vi "check_rs.vi"() -> ()   [LabVIEW 2013]
panel:
  in  "R&S address":string="29"
  out "address 2":string
  in  "amplitude (mV)":i32=10
  in  "modulation (kHz)":i32=100
  in  "center frequency (MHz)":dbl=32.7
  in  "exit":bool
  in  "rs_set":bool
  in  "rs_off":bool
  in  "rs_on":bool
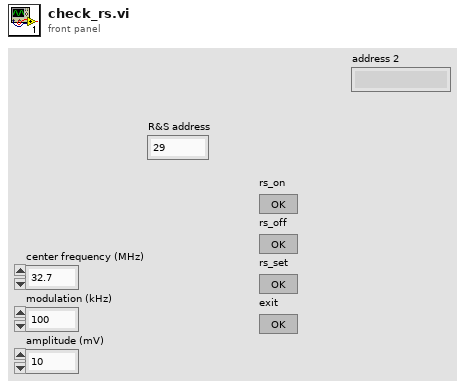
[diagram p1: front panel]
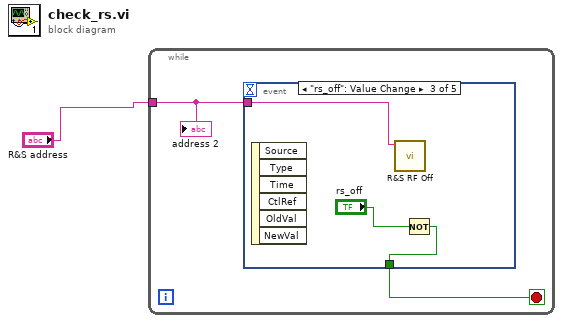
[diagram p0: block diagram]
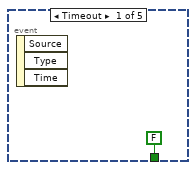
[diagram p2: hidden frame]
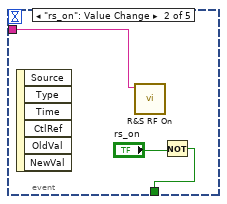
[diagram p3: hidden frame]
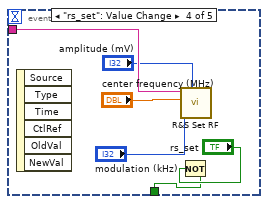
[diagram p4: hidden frame]
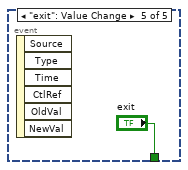
[diagram p5: hidden frame]
diagram:
  n1 = while {
    tunnel: "R&S address" -> [w2]
    stop <- w3 stop-if-true
    n2 = event shown="[2] \"rs_off\": Value Change" {
      selector: _ -> [_ _ _ _ _]
      dyn-events: _ -> [_ _ _ _ _]
      timeout: _ -> [_ _ _ _ _]
      tunnel: [FALSE ("exit") w5 w8 w11 "exit"] -> w3
      tunnel: w2 -> [_ w7 w10 w16 _]
      event Timeout {
        n3 = event-data() -> ()  [unwired: 1 in, 3 out]
      }
      event "rs_on": Value Change {
        n4 = event-data() -> ()  [unwired: 1 in, 6 out]
        n5 = call "R&S RF On.vi"("address"=w7) -> ()  [unwired: 5 in, 2 out]
        n6 = Not(x="rs_on") -> (.not. x?=w5:bool)
      }
      event "rs_off": Value Change {
        n7 = event-data() -> ()  [unwired: 1 in, 6 out]
        n8 = call "R&S RF Off.vi"("address"=w10) -> ()  [unwired: 5 in, 2 out]
        n9 = Not(x="rs_off") -> (.not. x?=w8:bool)
      }
      event "rs_set": Value Change {
        n10 = event-data() -> ()  [unwired: 1 in, 6 out]
        n11 = Not(x="rs_set") -> (.not. x?=w11:bool)
        n12 = call "R&S Set RF.vi"("amplitude (mV)"="amplitude (mV)", "modulation (kHz)"="modulation (kHz)", "center frequency (MHz)"="center frequency (MHz)", "address"=w16) -> ()  [unwired: 3 in, 2 out]
      }
      event "exit": Value Change {
        n13 = event-data() -> ()  [unwired: 1 in, 6 out]
      }
    }
    "address 2" <- w2
  }
